vi "GenerateSine.vi"(8 "amplitude":dbl=127.00000000000028 format="%0.2f", 9 "#samples":i32=989, 10 "FSsine_in":i32=96000, 11 "Cycles":i32=1) -> (2 "Array":dbl[](array[numeric]), 3 "Fsine_in":dbl=97.06774519716886)   [LabVIEW 2016]
uses:
  <vilib>/Analysis/NI_AALBase.lvlib
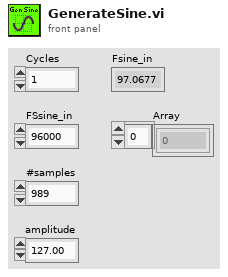
[diagram p1: front panel]
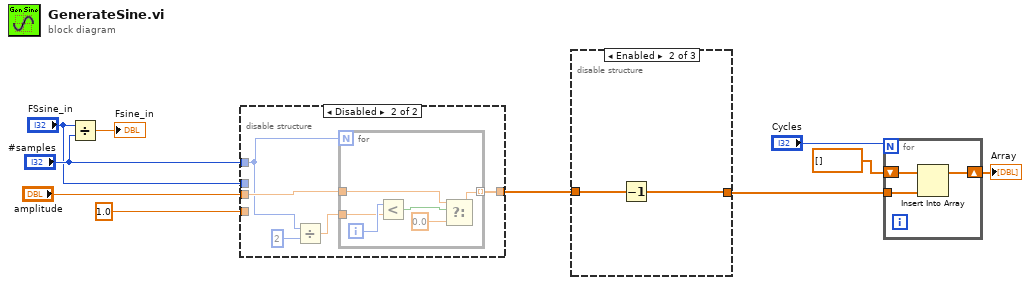
[diagram p0: block diagram]
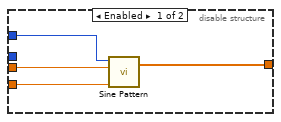
[diagram p2: hidden frame]
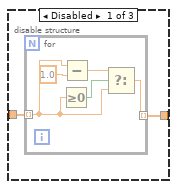
[diagram p3: hidden frame]
diagram:
  n1 = Divide(x="FSsine_in", y="#samples") -> (x/y=→"Fsine_in":dbl)
  n2 = disable-structure shown="Disabled" {
    disable-tunnel: "amplitude" -> [w14 w18]
    disable-tunnel: [w13 w19] -> w6
    disable-tunnel: 1.0 ("cycles") -> [w12 _]
    disable-tunnel: "#samples" -> [w11 w17]
    disable-tunnel: "FSsine_in" -> [_ _]
    frame Enabled {
      n3 = call <vilib>:"Sine Pattern.vi"("cycles"=w12, "amplitude"=w14, "samples"=w11) -> ("Sinusoidal Pattern"=w13:dbl[])  [unwired: 1 in, 1 out]
    }
    frame Disabled {
      n4 = Divide(x=w17, y=2) -> (x/y=w16:dbl)
      n5 = for {
        N: w17 -> [_]
        tunnel: [w24] -> w19 mode=indexing
        tunnel: w18 -> [w25]
        tunnel: w16 -> [w20]
        i -> [w22]
        n6 = Less?(x=w22, y=w20) -> (x < y?=w21:bool)
        n7 = Select(t=w25, s=w21, f=0.0) -> (s? t:f=w24:dbl)
      }
    }
  }
  n8 = disable-structure shown="Enabled" {
    disable-tunnel: [w27 w33 w35] -> w3
    disable-tunnel: w6 -> [w26 w34 w35]
    frame Disabled {
      n9 = for {
        tunnel: w26 -> [w31] mode=indexing
        tunnel: [w28] -> w27 mode=indexing
        n10 = Greater Or Equal To 0?(x=w31) -> (x >= 0?=w32:bool)
        n11 = Subtract(x=w31, y=1.0) -> (x-y=w30:dbl)
        n12 = Select(t=w30, s=w32, f=w31) -> (s? t:f=w28:dbl)
      }
    }
    frame Enabled {
      n13 = Decrement(x=w34) -> (x-1=w33:dbl[])
    }
    frame Disabled {
    }
  }
  n14 = for {
    N: "Cycles" -> [_]
    shift-right: [w37] -> w8
    shift-left: dbl[] [] -> [w38]
    tunnel: w3 -> [w36]
    n15 = Insert Into Array(array=w38, new element=w36) -> (w37:dbl[])  [unwired: 1 in]
  }
  "Array" <- w8
